vi "Update-acquisition-vars.vi"(8 "error in":errorcluster, 11 "Data ref. in":refnum<data-value>) -> (0 "error IO":errorcluster, 3 "Data ref.":refnum<data-value>, 4 "Image sizes":u32[][](array[numeric]), 6 "Camport array":u32[](array[numeric]))   [LabVIEW 2013, in "CameraVision.lvlib" / "CV-Main.lvclass"]
doc: "This function calculates some variables relaed to the number and order of the cameras and the size of each camera image. This information is later used to initialize the camera and image resources."
uses:
  CV-Main.lvclass
  CV-Main.lvclass/CV-Main.ctl
  Configuration/CV-Configuration.lvclass/CV-Configuration.ctl
  Storage/CV-Storage.lvclass/CV-Storage.ctl
  Read Config params.vi
  Read Storage params.vi
  Configuration/Read Camera 1 port.vi
  Configuration/Read Number of cameras.vi
  Configuration/Read ROI width.vi
  Configuration/Read ROI height.vi
  Storage/Write Camera suffix.vi
  Configuration/Write Camport array.vi
  Configuration/Write Image sizes.vi
  Configuration/Write Image arrays.vi
  Configuration/CV-Configuration.lvclass
  Storage/CV-Storage.lvclass
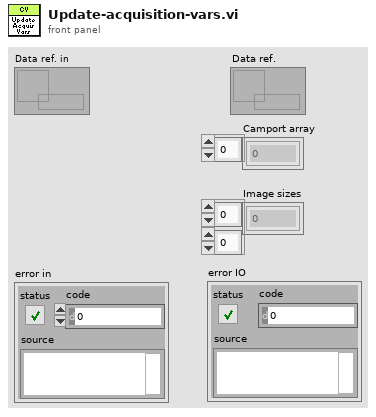
[diagram p1: front panel]
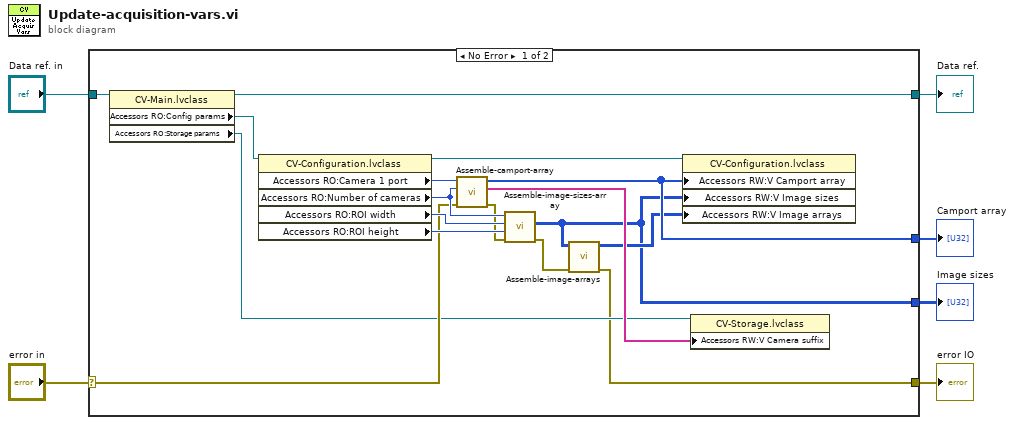
[diagram p0: block diagram]
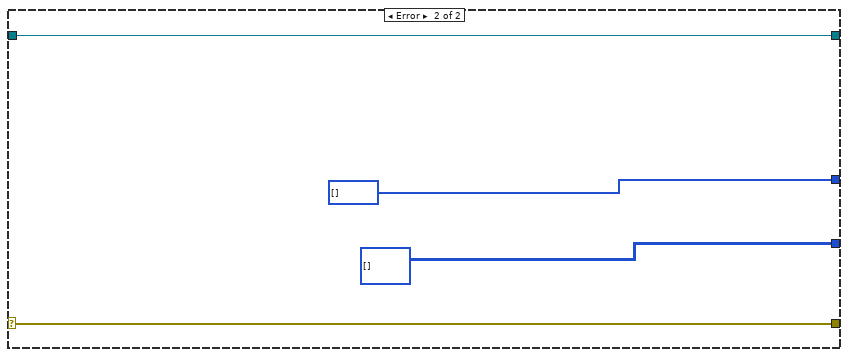
[diagram p2: hidden frame]
diagram:
  n1 = case shown="No Error" "error in" {
    selector: "error in" -> [w14 w25]
    tunnel: [w7 w25] -> w6
    tunnel: [w8 u32[][] [] ("Image sizes")] -> w5
    tunnel: [w17 u32[] [] ("Camport array")] -> w4
    tunnel: "Data ref. in" -> [w15 w24]
    tunnel: [w13 w24] -> w1
    frame No Error {
      n2 = property class="CV-Main.lvclass"(reference=w15) -> (reference out=w13:refnum<data-value>, "Accessors RO:Config params"=w12:refnum<data-value>, "Accessors RO:Storage params"=w11:refnum<data-value>)  [unwired: 1 in, 1 out]
      n3 = property class="CV-Configuration.lvclass"(reference=w12) -> (reference out=w18:refnum<data-value>, "Accessors RO:Camera 1 port"=w23:enum16{"A", "B"}, "Accessors RO:Number of cameras"=w22:i32, "Accessors RO:ROI width"=w21:u32, "Accessors RO:ROI height"=w20:u32)  [unwired: 1 in, 1 out]
      n4 = call "Assemble-camport-array.vi"("error in"=w14, "Number of cameras"=w22, "First camera port"=w23) -> ("error IO"=w19:errorcluster, "Camera suffix"=w16:string[], "Camport array"=w17:u32[])  [unwired: 6 in]
      n5 = call "Assemble-image-sizes-array.vi"("error in"=w19, "ROI height [pixels]"=w20, "ROI width [pixels]"=w21, "Number of cameras"=w22) -> ("error IO"=w10:errorcluster, "Image sizes"=w8:u32[][])  [unwired: 6 in]
      n6 = call "Assemble-image-arrays.vi"("error in"=w10, "Image sizes"=w8) -> ("error IO"=w7:errorcluster, "Zero images"=w9:i8[][][])  [unwired: 8 in]
      n7 = property class="CV-Configuration.lvclass"(reference=w18, "Accessors RW:V Camport array"=w17, "Accessors RW:V Image sizes"=w8, "Accessors RW:V Image arrays"=w9) -> ()  [unwired: 1 in, 2 out]
      n8 = property class="CV-Storage.lvclass"(reference=w11, "Accessors RW:V Camera suffix"=w16) -> ()  [unwired: 1 in, 2 out]
    }
    frame Error {
    }
  }
  "error IO" <- w6
  "Image sizes" <- w5
  "Camport array" <- w4
  "Data ref." <- w1
